vi "process_pixel_mapper_imaq_dll.vi"() -> ()   [LabVIEW 2011, in "Fiberscope_library.lvlib"]
uses:
  Fiberscope_library.lvlib
  typedefs/pixel_per_spiral_I32.ctl
  typedefs/image_size_I32.ctl
  typedefs/element_streams_cluster.ctl
  typedefs/control_process_state_cluster.ctl
  typedefs/control_process_state_enum.ctl
  typedefs/feedback_to_watchdog.ctl
  typedefs/feedback_from_process_enum.ctl
  typedefs/element_imaq_images_cluster.ctl
  <vilib>/vision/Image Controls.llb/IMAQ Image.ctl
  typedefs/all_scan_parameters_cluster.ctl
  typedefs/fiber_parameters_cluster.ctl
  fpga/typedefs/ramp_type_enum.ctl
  typedefs/spiral_parameters_cluster.ctl
  typedefs/run_parameters_cluster.ctl
  typedefs/run_mode_enum.ctl
  typedefs/acquisition_parameters_cluster.ctl
  typedefs/smooth_coeffs_cluster.ctl
  typedefs/storage_parameters_cluster.ctl
  typedefs/mapping_corrections_cluster.ctl
  typedefs/pockels_corrections_cluster.ctl
  Fiberscope_support_dll/Debug/Fiberscope_support_dll.dll
panel:
  out "Phase corrections":dbl[][](graph)
  out "Amplitude corrections":dbl[][](graph)
  out "Local_exit":bool
  out "Pixelhits":dbl[][](graph)
  out "Pixel map":cluster{i32[], i32[]}(graph)
  out "error out":errorcluster
  in  "error in":errorcluster
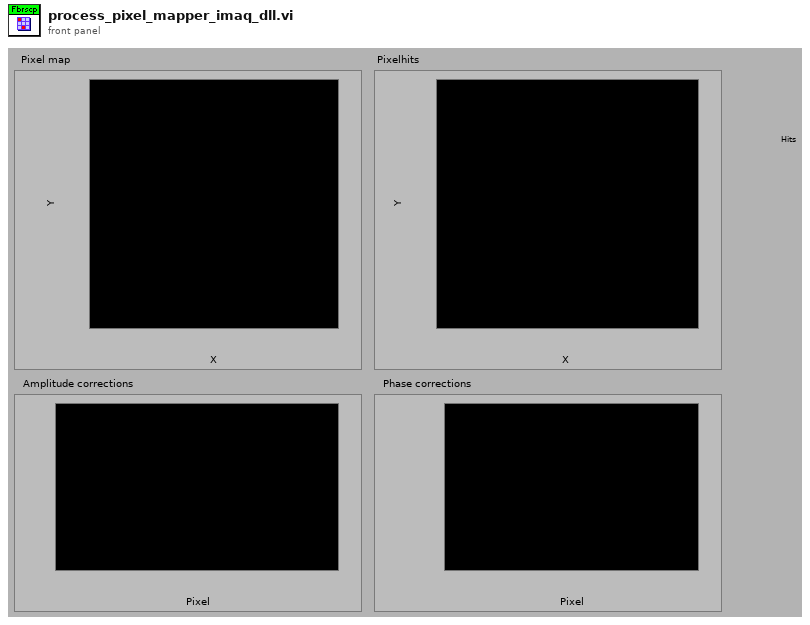
[diagram p1: front panel]
types:
  T1 = typedef "Fiberscope_library.lvlib/feedback_to_watchdog.ctl" = cluster{"Feedback_from_process_enum":T2, "Process_name":string}
  T2 = typedef "Fiberscope_library.lvlib/feedback_from_process_enum.ctl" = enum16{"Has_initialised", "Changed_parameters", "Has_started", "Has_stopped", "Has_quitted", "Is_running", "Has_finished", "Custom"}
  T3 = typedef "Fiberscope_library.lvlib/control_process_state_cluster.ctl" = cluster{"Control_process_state_enum":T4, "variant":variant}
  T4 = typedef "Fiberscope_library.lvlib/control_process_state_enum.ctl" = enum16{"Init", "Quit", "Start", "Stop", "Change_parameters", "Running", "Finish", "Custom"}
  T5 = typedef "Fiberscope_library.lvlib/element_streams_cluster.ctl" = cluster{"Streams_array":dbl[][], "#channels":i32, "Last element?":bool, "Forth (1) or back (0)?":bool}
  T6 = typedef "Fiberscope_library.lvlib/image_size_I32.ctl" = i32
  T7 = typedef "Fiberscope_library.lvlib/pixel_per_spiral_I32.ctl" = i32
  T8 = typedef "Fiberscope_library.lvlib/element_imaq_images_cluster.ctl" = cluster{"Images":T9[], "#channels":i32, "Last element?":bool}
  T9 = typedef "IMAQ Image.ctl" = refnum<image>
  T10 = typedef "Fiberscope_library.lvlib/all_scan_parameters_cluster.ctl" = cluster{"Fiber parameters":T11, "Spiral parameters":T13, "Run parameters":T14, "Acquisition parameters":T16, "Fiber parameters pixel_mapper":T11, "Smooth_coeffs_cluster":T17, "Storage parameters":T18, "Mapping corrections":T19, "Pockels corrections":T20}
  T11 = typedef "Fiberscope_library.lvlib/fiber_parameters_cluster.ctl" = cluster{"Frequency":dbl, "Amplitude X":dbl, "Amplitude Y":dbl, "Initial Amplitude X":dbl, "Initial Amplitude Y":dbl, "Phase":dbl, "Ramp type":T12}
  T12 = typedef "ramp_type_enum.ctl" = enum8{"Linear", "Sine"}
  T13 = typedef "Fiberscope_library.lvlib/spiral_parameters_cluster.ctl" = cluster{"Imaging periods":dbl, "Settling periods":dbl, "Resting periods":dbl}
  T14 = typedef "Fiberscope_library.lvlib/run_parameters_cluster.ctl" = cluster{"Run mode":T15, "Averages per frame":u8, "No. of frames":u32}
  T15 = typedef "Fiberscope_library.lvlib/run_mode_enum.ctl" = enum16{"Continuous", "Single frame", "No. of frames"}
  T16 = typedef "Fiberscope_library.lvlib/acquisition_parameters_cluster.ctl" = cluster{"Cycles per pixel":u32, "Image size":T6, "Bidirectional acquisition":bool}
  T17 = typedef "Fiberscope_library.lvlib/smooth_coeffs_cluster.ctl" = cluster{"Coeff 1":dbl, "Coeff 2":dbl}
  T18 = typedef "Fiberscope_library.lvlib/storage_parameters_cluster.ctl" = cluster{"Autosave":bool, "Path":path}
  T19 = typedef "Fiberscope_library.lvlib/mapping_corrections_cluster.ctl" = cluster{"Phase increase":dbl, "Amplitude correction":dbl}
  T20 = typedef "Fiberscope_library.lvlib/pockels_corrections_cluster.ctl" = cluster{"Delay pixels":i32}
  T21 = typedef "Fiberscope_library.lvlib/lookup_arrays_ref_cluster.ctl" = cluster{"rows":refnum<data-value>, "cols":refnum<data-value>}
  T22 = typedef "Image Type" = u32
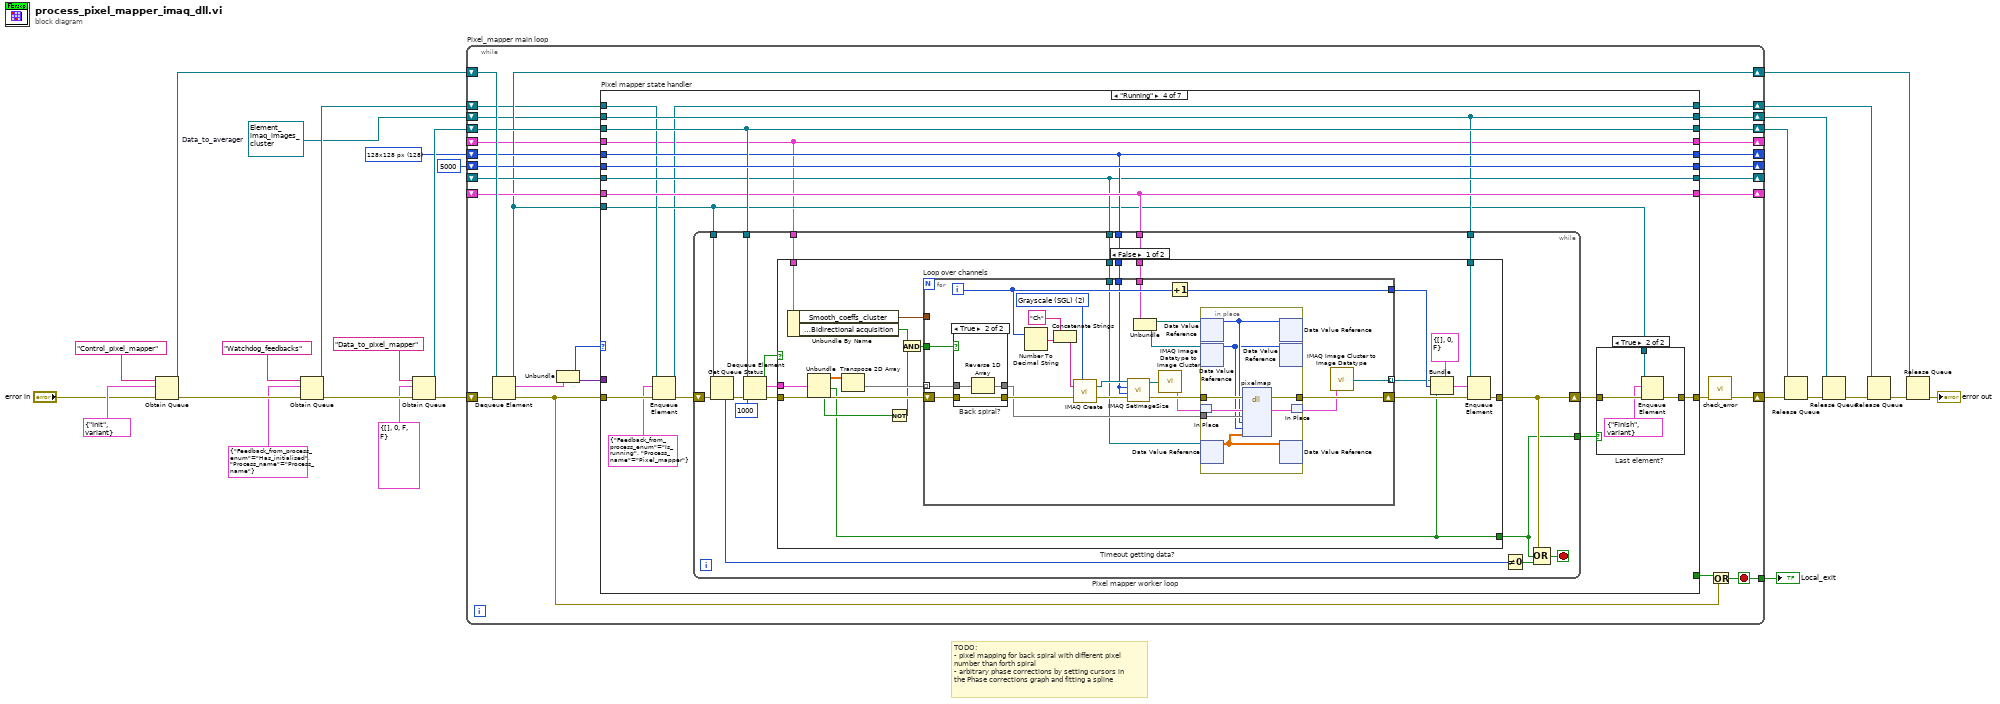
[diagram p0: block diagram]
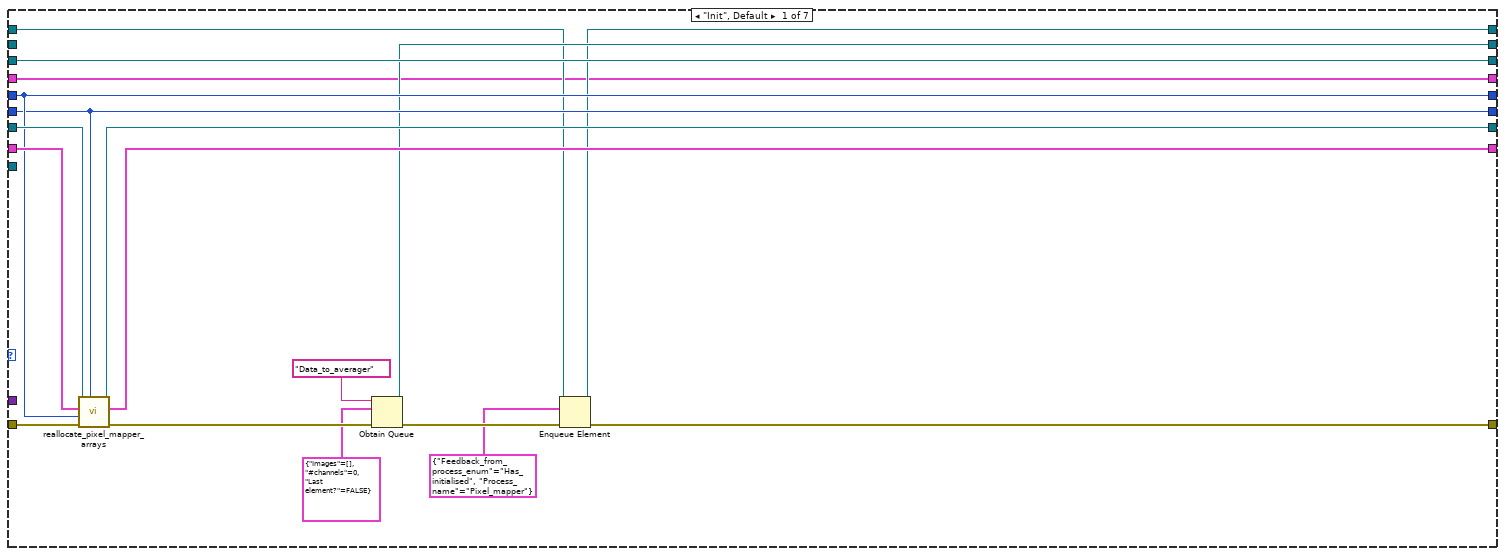
[diagram p2: hidden frame]
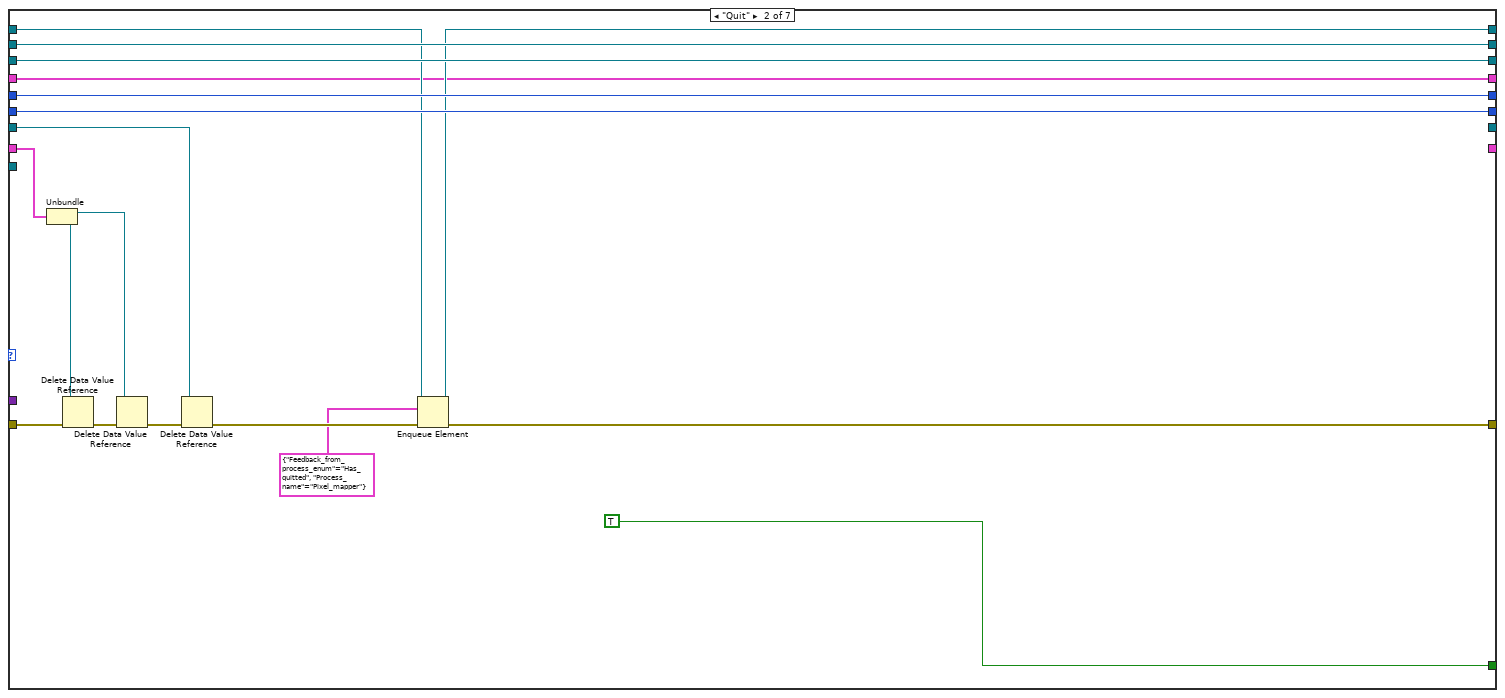
[diagram p3: hidden frame]
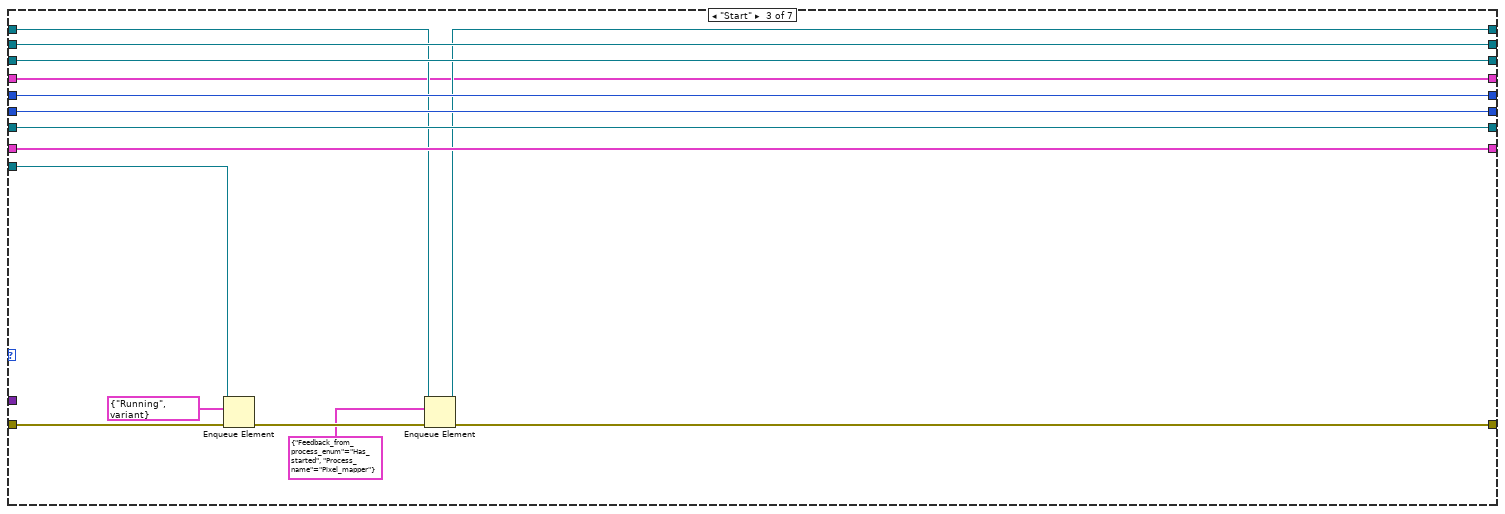
[diagram p4: hidden frame]
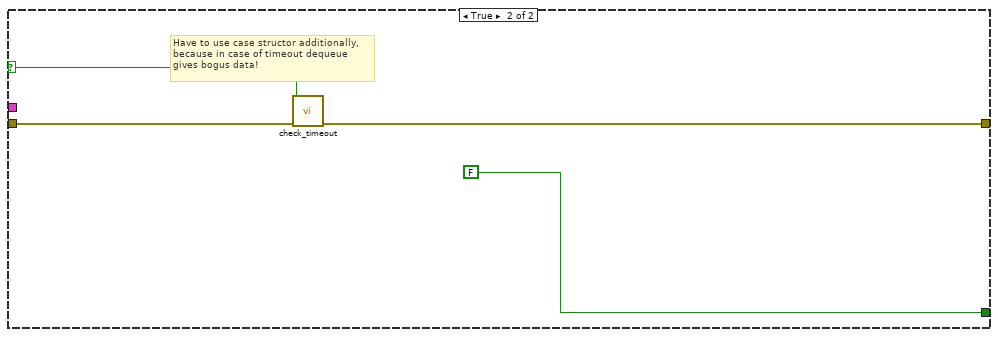
[diagram p7: hidden frame]
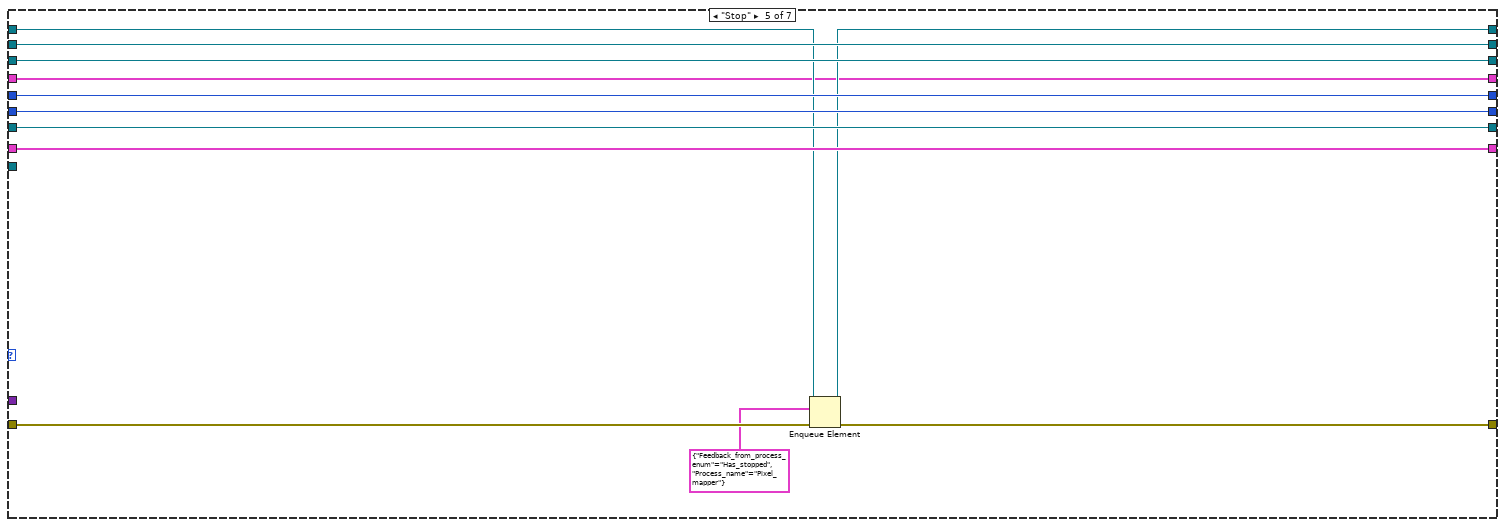
[diagram p8: hidden frame]
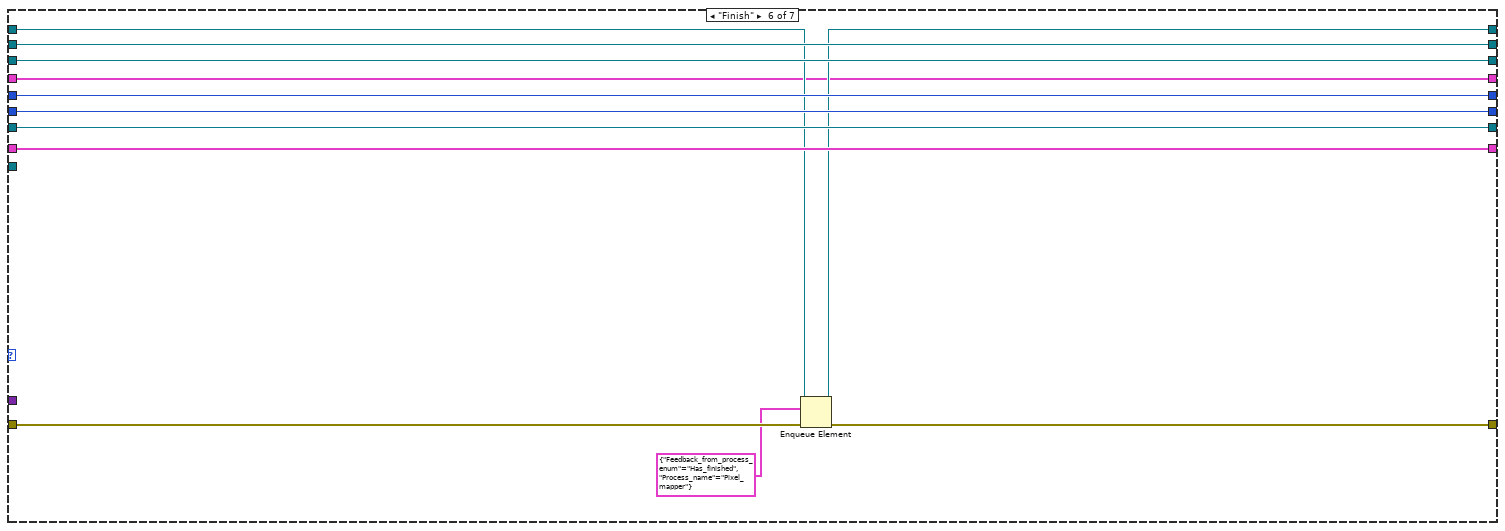
[diagram p9: hidden frame]
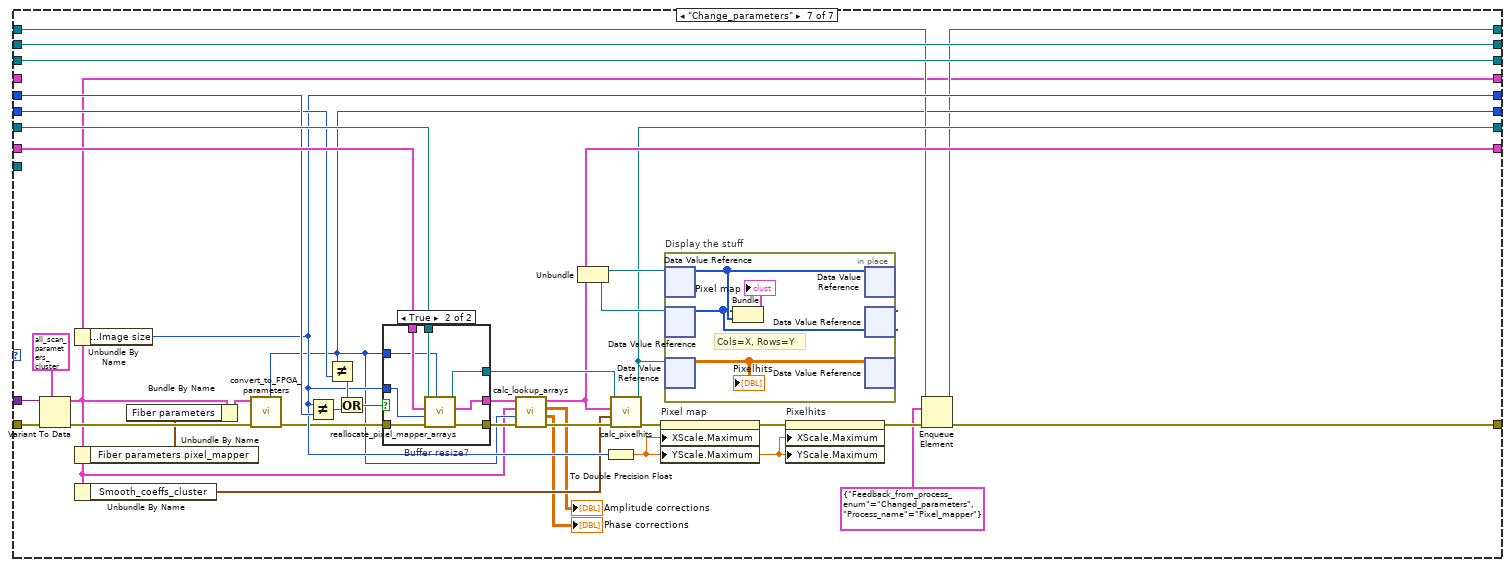
[diagram p10: hidden frame]
diagram:
  w1 = refnum<queue> refnum  # Data_to_averager
  w17 = T6 128 items=["128x128 px"=128, "256x256 px"=256, "512x512 px"=512] ("Image size")
  # "TODO:\n- pixel mapping for back spiral with different pixel\nnumber than forth spiral\n- arbitrary phase corrections by setting cursors in \nthe Phase corrections graph and fitting a spline"
  n1 = Obtain Queue(name (unnamed)="Control_pixel_mapper", element data type=T3 {"Control_process_state_enum"=enum."Init", "variant"=variant} ("Control_process_state_cluster"), error in (no error)="error in") -> (queue out=w2:refnum<queue>, error out=w16:errorcluster)  [unwired: 2 in, 1 out]
  n2 = Obtain Queue(name (unnamed)="Watchdog_feedbacks", element data type=T1 {"Feedback_from_process_enum"=enum."Has_initialised", "Process_name"="Process_name"}, error in (no error)=w16) -> (queue out=w13:refnum<queue>, error out=w15:errorcluster)  [unwired: 2 in, 1 out]
  n3 = Obtain Queue(name (unnamed)="Data_to_pixel_mapper", element data type=T5 {"Streams_array"=[], "#channels"=0, "Last element?"=FALSE, "Forth (1) or back (0)?"=FALSE} ("Element_from_DAQ_cluster"), error in (no error)=w15) -> (queue out=w21:refnum<queue>, error out=w23:errorcluster)  [unwired: 2 in, 1 out]
  n4 = while "Pixel_mapper main loop" {
    shift-right: [w47] -> w20
    shift-left: w23 -> [w53]
    shift-right: [w39] -> _
    shift-left: w17 -> [w44]
    shift-right: [w43] -> _
    shift-left: _ -> [w42]
    shift-right: [w41] -> _
    shift-left: _ -> [w40]
    shift-right: [w37] -> _
    shift-left: T7 5000 ("Pixels per spiral") -> [w38]
    shift-right: [w34] -> w8
    shift-left: w1 -> [w35]
    shift-right: [w36] -> w24
    shift-left: w2 -> [w52]
    shift-right: [w45] -> w19
    shift-left: w21 -> [w46]
    shift-right: [w32] -> w11
    shift-left: w13 -> [w33]
    tunnel: [w29] -> w3
    shift-right: [w28] -> _
    shift-left: _ -> [w27]
    stop <- w29 stop-if-true
    n5 = Dequeue Element(queue=w52, error in (no error)=w53) -> (queue out=w36:refnum<queue>, element=w51:T3, error out=w30:errorcluster)  [unwired: 1 in, 1 out]
    n6 = Unbundle(w51) -> ("Control_process_state_enum"=w49:T4, "variant"=w50:variant)
    n7 = case "Pixel mapper state handler" shown="\"Running\"" w49 {
      tunnel: w30 -> [w70 w86 w96 w114 w211 w223 w266]
      tunnel: [w59 w76 w94 w110 w210 w222 w243] -> w48
      tunnel: w50 -> [_ _ _ _ _ _ w265]
      tunnel: w46 -> [w71 w89 w103 w119 w217 w229 w267]
      tunnel: [w71 w89 w103 w119 w217 w229 w267] -> w45
      tunnel: w44 -> [w65 w88 w101 w117 w214 w226 w253]
      tunnel: [w66 _ w100 w116 w216 w228 w254] -> w43
      tunnel: w42 -> [w68 w82 w100 w116 w216 w228 w261]
      tunnel: [w67 _ w102 w118 w215 w227 w257] -> w41
      tunnel: w40 -> [w69 w87 w102 w118 w215 w227 w262]
      tunnel: [w65 w88 w101 w117 w214 w226 w245] -> w39
      tunnel: w38 -> [w62 w80 w104 w120 w213 w225 w249]
      tunnel: [w62 w80 w104 w120 w213 w225 w238] -> w37
      tunnel: w36 -> [_ _ w97 w108 _ _ _]
      tunnel: w35 -> [_ w79 w99 w115 w212 w224 w258]
      tunnel: [_ TRUE _ _ _ _ _] -> w31
      tunnel: [w61 w79 w99 w115 w212 w224 w258] -> w34
      tunnel: w33 -> [w58 w75 w98 w112 w209 w221 w242]
      tunnel: [w57 w74 w92 w107 w208 w220 w237] -> w32
      tunnel: [w55 w72 w90 w105 w206 w218 w234] -> w28
      tunnel: w27 -> [w55 w72 w90 w105 w206 w218 _]
      frame "Init", Default {
        n8 = call "reallocate_pixel_mapper_arrays.vi"("New pixels per spiral"=w62, "error in"=w70, "New image size"=w65, "Lookup arrays in"=w69, "Pixelhits array in"=w68) -> ("error out"=w64:errorcluster, "Lookup arrays out"=w67:T21, "Pixelhits array out"=w66:refnum<data-value>)  [unwired: 4 in]
        n9 = Obtain Queue(name (unnamed)="Data_to_averager", element data type=T8 {"Images"=[], "#channels"=0, "Last element?"=FALSE} ("Element_imaq_images_cluster"), error in (no error)=w64) -> (queue out=w61:refnum<queue>, error out=w60:errorcluster)  [unwired: 2 in, 1 out]
        n10 = Enqueue Element(queue=w58, element=T1 {"Feedback_from_process_enum"=enum."Has_initialised", "Process_name"="Pixel_mapper"}, error in (no error)=w60) -> (queue out=w57:refnum<queue>, error out=w59:errorcluster)  [unwired: 1 in, 1 out]
      }
      frame "Quit" {
        n11 = Unbundle(w87) -> ("rows"=w83:refnum<data-value>, "cols"=w85:refnum<data-value>)
        n12 = Delete Data Value Reference(data value reference=w85, error in=w86) -> (error out=w84:errorcluster)  [unwired: 1 out]
        n13 = Delete Data Value Reference(data value reference=w83, error in=w84) -> (error out=w81:errorcluster)  [unwired: 1 out]
        n14 = Delete Data Value Reference(data value reference=w82, error in=w81) -> (error out=w77:errorcluster)  [unwired: 1 out]
        n15 = Enqueue Element(queue=w75, element=T1 {"Feedback_from_process_enum"=enum."Has_quitted", "Process_name"="Pixel_mapper"}, error in (no error)=w77) -> (queue out=w74:refnum<queue>, error out=w76:errorcluster)  [unwired: 1 in, 1 out]
      }
      frame "Start" {
        n16 = Enqueue Element(queue=w97, element=T3 {"Control_process_state_enum"=enum."Running", "variant"=variant} ("Control_process_state_cluster"), error in (no error)=w96) -> (error out=w95:errorcluster)  [unwired: 1 in, 2 out]
        n17 = Enqueue Element(queue=w98, element=T1 {"Feedback_from_process_enum"=enum."Has_started", "Process_name"="Pixel_mapper"}, error in (no error)=w95) -> (queue out=w92:refnum<queue>, error out=w94:errorcluster)  [unwired: 1 in, 1 out]
      }
      frame "Running" {
        n18 = Enqueue Element(queue=w112, element=T1 {"Feedback_from_process_enum"=enum."Is_running", "Process_name"="Pixel_mapper"}, error in (no error)=w114) -> (queue out=w107:refnum<queue>, error out=w113:errorcluster)  [unwired: 1 in, 1 out]
        n19 = while "Pixel mapper worker loop" {
          shift-right: [w130] -> w111
          shift-left: w113 -> [w138]
          tunnel: w119 -> [w143]
          tunnel: w108 -> [w139]
          tunnel: w115 -> [w136]
          tunnel: w118 -> [w133]
          tunnel: w117 -> [w132]
          tunnel: w116 -> [w131]
          tunnel: [w127] -> w109
          tunnel: w105 -> [w126]
          stop <- w140 stop-if-true
          n20 = Get Queue Status(queue=w139, error in (no error)=w138) -> (error out=w137:errorcluster, # elements in queue=w142:i32)  [unwired: 1 in, 6 out]
          n21 = Dequeue Element(queue=w143, timeout in ms (-1)=1000, error in (no error)=w137) -> (element=w128:T5, timed out?=w134:bool, error out=w129:errorcluster)  [unwired: 1 out]
          n22 = case "Timeout getting data?" shown="False" w134 {
            selector: w134 -> [_ w203]
            tunnel: w129 -> [w162 w205]
            tunnel: [w164 w204] -> w130
            tunnel: w136 -> [w163 _]
            tunnel: w128 -> [w159 _]
            tunnel: w133 -> [w146 _]
            tunnel: w132 -> [w151 _]
            tunnel: w131 -> [w145 _]
            tunnel: [w147 FALSE ("Last element?")] -> w127
            tunnel: w126 -> [w157 _]
            frame False {
              n23 = Unbundle By Name(w157) -> ("Smooth_coeffs_cluster"=w156:T17, "Acquisition parameters.Bidirectional acquisition"=w153:bool)
              n24 = Unbundle(w159) -> ("Streams_array"=w160:dbl[][], "Last element?"=w147:bool, "Forth (1) or back (0)?"=w154:bool)  [unwired: 1 out]
              n25 = Transpose 2D Array(2D array=w160) -> (transposed array=w158:dbl[][])
              n26 = Not(x=w154) -> (.not. x?=w155:bool)
              n27 = And(x=w153, y=w155) -> (x .and. y?=w152:bool)
              n28 = for "Loop over channels" {
                tunnel: w158 -> [w186] mode=indexing
                shift-right: [w174] -> w161
                shift-left: w162 -> [w187]
                tunnel: [w188] -> w148
                tunnel: w156 -> [_]
                tunnel: w152 -> [w185]
                tunnel: w151 -> [w176]
                tunnel: w146 -> [w171]
                tunnel: w145 -> [w167]
                tunnel: [w165] -> w144 mode=indexing
                i -> [w183]
                w179 = T22 2 items=["Grayscale (U8)", "Grayscale (I16)", "Grayscale (SGL)", "Complex (CSG)", "RGB (U32)", "HSL (U32)", "RGB (U64)", "Grayscale (U16)"] ("Image Type")
                n29 = case "Back spiral?" shown="True" w185 {
                  tunnel: w187 -> [w197 w201]
                  tunnel: [w197 w201] -> w184
                  tunnel: w186 -> [w198 w200]
                  tunnel: [w198 w199] -> w172
                  frame False {
                  }
                  frame True {
                    n30 = Reverse 1D Array(array=w200) -> (reversed array=w199:dbl[])
                  }
                }
                n31 = Number To Decimal String(number=w183) -> (decimal integer string=w181:string)  [unwired: 1 in]
                n32 = Concatenate Strings("Ch" ("Image Name"), w181) -> (w180:string)
                n33 = call "IMAQ Create"("Image Name"=w180, "Image Type"=w179, "error in (no error)"=w184) -> ("New Image"=w177:T9, "error out"=w178:errorcluster)  [unwired: 2 in]
                n34 = call "IMAQ SetImageSize"("error in (no error)"=w178, "Y Resolution"=w176, "X Resolution"=w176, "Image"=w177) -> ("error out"=w175:errorcluster, "Image Out"=w173:T9)  [unwired: 1 in]
                n35 = Unbundle(w171) -> ("rows"=w169:refnum<data-value>, "cols"=w168:refnum<data-value>)
                n36 = call <vilib>:"IMAQ Image Datatype to Image Cluster.vi"("Image"=w173) -> ("Image (dup)"=w170:cluster{string, u32})
                n37 = Increment(x=w183) -> (x+1=w188:i32)
                n38 = in-place {
                  in-place-border: w175 -> [w196]
                  in-place-border: [w195] -> w174
                  in-place-border: w172 -> [w194]
                  n39 = in-place-dvr #1(w169) -> (w192:i32[])  [unwired: 1 out]
                  n40 = in-place-dvr #2(w168) -> (w191:i32[])  [unwired: 1 out]
                  n41 = in-place-match #3(w170) -> (w193:cluster{string, u32})
                  n42 = in-place-dvr #4(w167) -> (w190:dbl[][])  [unwired: 1 out]
                  n43 = dll-call lib="C:/helioscan/tools/Fiberscope_RK110722/Fiberscope_support_dll/Debug/Fiberscope_support_dll.dll" fn="pixelmap"(error in=w196, "LVImage"=w193, "adRawdata"=w194, "aiLookupX"=w192, "aiLookupY"=w191, "aiPixelhits"=w190) -> (error out=w195:errorcluster, "LVImage"=w189:cluster{string, u32})  [unwired: 7 in, 1 out]
                  n44 = in-place-dvr #1(w192) -> ()  [unwired: 2 out]
                  n45 = in-place-dvr #2(w191) -> ()  [unwired: 2 out]
                  n46 = in-place-dvr #4(w190) -> ()  [unwired: 2 out]
                  n47 = in-place-match #3(w189) -> (w166:cluster{string, u32})
                }
                n48 = call <vilib>:"IMAQ Image Cluster to Image Datatype.vi"("Image"=w166) -> ("Image (dup)"=w165:T9)
              }
              n49 = Bundle(cluster=T8 {"Images"=[], "#channels"=0, "Last element?"=FALSE} ("Element_imaq_images_cluster"), "Images"=w144, "#channels"=w148, "Last element?"=w147) -> (w149:T8)
              n50 = Enqueue Element(queue=w163, element=w149, error in (no error)=w161) -> (error out=w164:errorcluster)  [unwired: 1 in, 2 out]
            }
            frame True {
              # "Have to use case structor additionally,\nbecause in case of timeout dequeue\ngives bogus data!"
              n51 = call "check_timeout.vi"("error in"=w205, "Timeout?"=w203) -> ("error out"=w204:errorcluster)  [unwired: 9 in]
            }
          }
          n52 = Not Equal To 0?(x=w142) -> (x != 0?=w141:bool)
          n53 = Compound Arithmetic op=OR(w130, w127, w141) -> (w140:bool)
        }
        n54 = case "Last element?" shown="True" w109 {
          tunnel: w111 -> [w121 w125]
          tunnel: [w121 w124] -> w110
          tunnel: w108 -> [_ w123]
          frame False {
          }
          frame True {
            n55 = Enqueue Element(queue=w123, element=T3 {"Control_process_state_enum"=enum."Finish", "variant"=variant} ("Control_process_state_cluster"), error in (no error)=w125) -> (error out=w124:errorcluster)  [unwired: 1 in, 2 out]
          }
        }
      }
      frame "Stop" {
        n56 = Enqueue Element(queue=w209, element=T1 {"Feedback_from_process_enum"=enum."Has_stopped", "Process_name"="Pixel_mapper"}, error in (no error)=w211) -> (queue out=w208:refnum<queue>, error out=w210:errorcluster)  [unwired: 1 in, 1 out]
      }
      frame "Finish" {
        n57 = Enqueue Element(queue=w221, element=T1 {"Feedback_from_process_enum"=enum."Has_finished", "Process_name"="Pixel_mapper"}, error in (no error)=w223) -> (queue out=w220:refnum<queue>, error out=w222:errorcluster)  [unwired: 1 in, 1 out]
      }
      frame "Change_parameters" {
        n58 = Variant To Data(error in=w266, type=T10 {"Fiber parameters"={"Frequency"=100.0, "Amplitude X"=0.0, "Amplitude Y"=0.0, "Initial Amplitude X"=0.0, "Initial Amplitude Y"=0.0, "Phase"=0.0, "Ramp type"=enum."Linear"}, "Spiral parameters"={"Imaging periods"=1.0, "Settling periods"=1.0, "Resting periods"=1.0}, "Run parameters"={"Run mode"=enum."Continuous", "Averages per frame"=0, "No. of frames"=0}, "Acquisition parameters"={"Cycles per pixel"=0, "Image size"=1, "Bidirectional acquisition"=FALSE}, "Fiber parameters pixel_mapper"={"Frequency"=0.0, "Amplitude X"=0.0, "Amplitude Y"=0.0, "Initial Amplitude X"=0.0, "Initial Amplitude Y"=0.0, "Phase"=0.0, "Ramp type"=enum."Linear"}, "Smooth_coeffs_cluster"={"Coeff 1"=0.0, "Coeff 2"=0.0}, "Storage parameters"={"Autosave"=FALSE, "Path"=path ""}, "Mapping corrections"={"Phase increase"=0.0, "Amplitude correction"=0.0}, "Pockels corrections"={"Delay pixels"=0}} ("All scan parameters"), Variant=w265) -> (data=w234:T10, error out=w240:errorcluster)
        n59 = Unbundle By Name(w234) -> ("Acquisition parameters.Image size"=w245:T6)
        n60 = Unbundle By Name(w234) -> ("Fiber parameters pixel_mapper"=w232:T11)
        n61 = Unbundle By Name(w234) -> ("Smooth_coeffs_cluster"=w235:T17)
        n62 = Bundle By Name(cluster=w234, "Fiber parameters"=w232) -> (w233:T10)
        n63 = call "convert_to_FPGA_parameters.vi"("error in"=w240, "All scan parameters"=w233) -> ("error out"=w239:errorcluster, "Pixels per spiral"=w238:i32)  [unwired: 4 in, 4 out]
        n64 = Not Equal?(x=w245, y=w253) -> (x != y?=w251:bool)
        n65 = Not Equal?(x=w238, y=w249) -> (x != y?=w252:bool)
        n66 = Or(x=w252, y=w251) -> (x .or. y?=w250:bool)
        n67 = case "Buffer resize?" shown="True" w250 {
          tunnel: w239 -> [w274 w282]
          tunnel: [w274 w281] -> w263
          tunnel: w262 -> [w273 w279]
          tunnel: w261 -> [w272 w278]
          tunnel: [w273 w277] -> w260
          tunnel: [w272 w276] -> w259
          tunnel: w245 -> [_ w280]
          tunnel: w238 -> [_ w275]
          frame False {
          }
          frame True {
            n68 = call "reallocate_pixel_mapper_arrays.vi"("New pixels per spiral"=w275, "error in"=w282, "New image size"=w280, "Lookup arrays in"=w279, "Pixelhits array in"=w278) -> ("error out"=w281:errorcluster, "Lookup arrays out"=w277:T21, "Pixelhits array out"=w276:refnum<data-value>)  [unwired: 4 in]
          }
        }
        n69 = call "calc_lookup_arrays.vi"("error in"=w263, "Pixels per spiral"=w238, "All scan parameters"=w234, "Lookup arrays in"=w260) -> ("error out"=w264:errorcluster, "Phase corrections"=→"Phase corrections":dbl[][], "Amplitude corrections"=→"Amplitude corrections":dbl[][], "Lookup arrays out"=w257:T21)  [unwired: 4 in]
        n70 = Unbundle(w257) -> ("rows"=w256:refnum<data-value>, "cols"=w255:refnum<data-value>)
        n71 = To Double Precision Float(number=w245) -> (double precision float=w246:dbl)
        n72 = call "calc_pixelhits.vi"("error in"=w264, "Smooth_coeffs_cluster"=w235, "Lookup arrays"=w257, "Pixelhits array in"=w259) -> ("error out"=w248:errorcluster, "Pixelhits array out"=w254:refnum<data-value>)  [unwired: 6 in]
        n73 = property on="Pixel map" class="XYGraph (strict)"(error in=w248, "XScale.Maximum"=w246, "YScale.Maximum"=w246) -> (error out=w247:errorcluster)  [unwired: 1 in, 1 out]
        n74 = in-place "Display the stuff" {
          # "Cols=X, Rows=Y"
          n75 = in-place-dvr #5(w256) -> (w271:i32[])  [unwired: 1 out]
          n76 = in-place-dvr #6(w255) -> (w270:i32[])  [unwired: 1 out]
          n77 = in-place-dvr #7(w254) -> (w268:dbl[][])  [unwired: 1 out]
          "Pixelhits" <- w268
          n78 = Bundle(w270, w271) -> (→"Pixel map":cluster{i32[], i32[]})  [unwired: 1 in]
          n79 = in-place-dvr #5(w271) -> ()  [unwired: 2 out]
          n80 = in-place-dvr #6(w270) -> ()  [unwired: 2 out]
          n81 = in-place-dvr #7(w268) -> ()  [unwired: 2 out]
        }
        n82 = property on="Pixelhits" class="IntGraph (strict)"(error in=w247, "XScale.Maximum"=w246, "YScale.Maximum"=w246) -> (error out=w244:errorcluster)  [unwired: 1 in, 1 out]
        n83 = Enqueue Element(queue=w242, element=T1 {"Feedback_from_process_enum"=enum."Changed_parameters", "Process_name"="Pixel_mapper"}, error in (no error)=w244) -> (queue out=w237:refnum<queue>, error out=w243:errorcluster)  [unwired: 1 in, 1 out]
      }
    }
    n84 = call "check_error.vi"("error in"=w48) -> ("error out"=w47:errorcluster)  [unwired: 10 in]
    n85 = Or(x=w31, y=w30) -> (x .or. y?=w29:bool)
  }
  "Local_exit" <- w3
  n86 = Release Queue(queue=w19, error in (no error)=w20) -> (error out=w10:errorcluster)  [unwired: 1 in, 2 out]
  n87 = Release Queue(queue=w8, error in (no error)=w10) -> (error out=w9:errorcluster)  [unwired: 1 in, 2 out]
  n88 = Release Queue(queue=w11, error in (no error)=w9) -> (error out=w12:errorcluster)  [unwired: 1 in, 2 out]
  n89 = Release Queue(queue=w24, error in (no error)=w12) -> (error out=→"error out":errorcluster)  [unwired: 1 in, 2 out]
